vi "Section Page.vi"(8 "error in (no error)":errorcluster, 11 "Node Ptr":T1 format="%.0x") -> (0 "error out":errorcluster)   [LabVIEW 2023, in "J1939 Addon System Explorer.lvlib"]
uses:
  J1939 Addon System Explorer.lvlib
  <vilib>/NI VeriStand/Custom Device API/Custom Device Item Ref.ctl
  Addon Shared/SubVIs/Constants.vi
  <vilib>/NI VeriStand/Custom Device API/Custom Device API.lvlib
  Addon Shared/J1939 Addon Shared.lvlib
panel:
  in  "SHDocVw.IWebBrowser2":refnum<k7>(container)
types:
  T1 = typedef "Custom Device API.lvlib/Custom Device Item Ref.ctl" = u64
  T2 = typedef "Custom Device API.lvlib/Custom Device Item Info.ctl" = cluster{"Name":string, "Is Channel":bool, "GUID":string, "Is Waveform":bool}
  T3 = typedef "Custom Device API.lvlib/Custom Device Commands.ctl" = enum16{"Default", "Item renamed", "Shutdown", "Dynamic button pressed"}
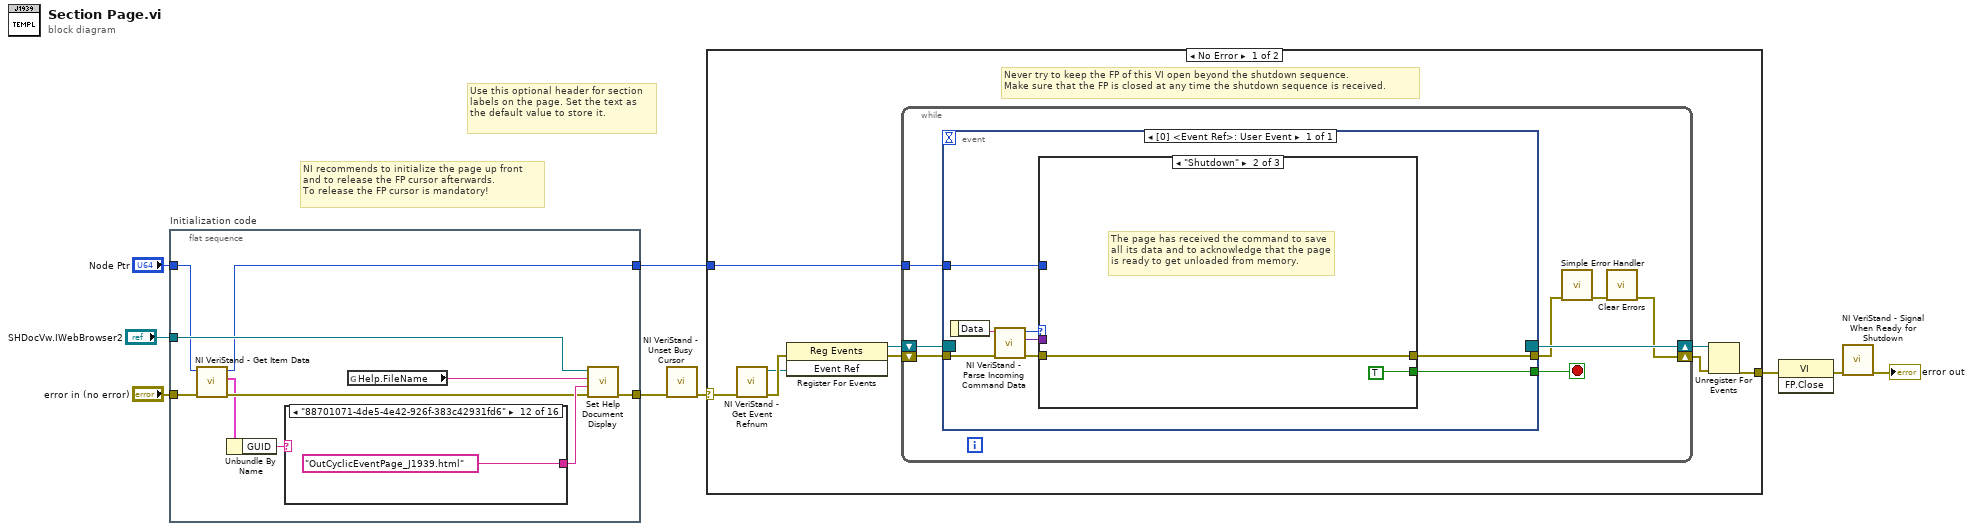
[diagram p0: block diagram]
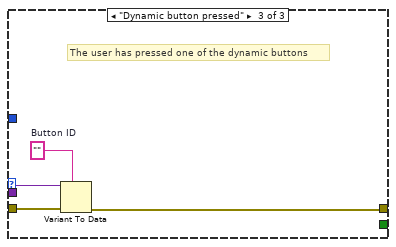
[diagram p3: hidden frame]
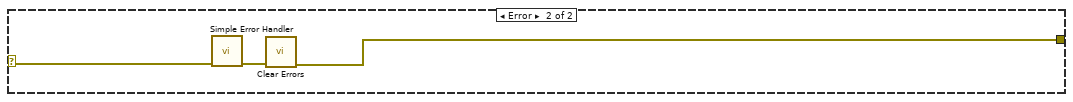
[diagram p4: hidden frame]
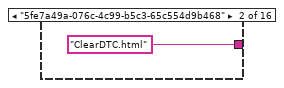
[diagram p6: hidden frame]
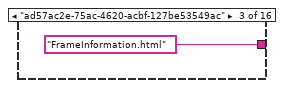
[diagram p7: hidden frame]
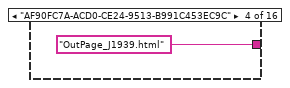
[diagram p8: hidden frame]
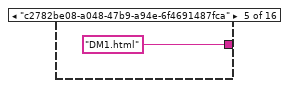
[diagram p9: hidden frame]
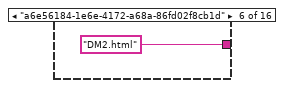
[diagram p10: hidden frame]
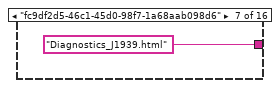
[diagram p11: hidden frame]
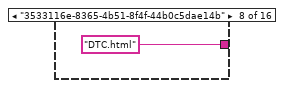
[diagram p12: hidden frame]
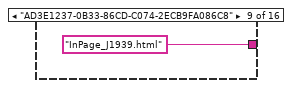
[diagram p13: hidden frame]
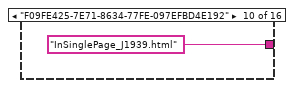
[diagram p14: hidden frame]
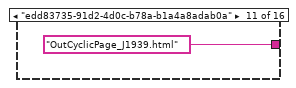
[diagram p15: hidden frame]
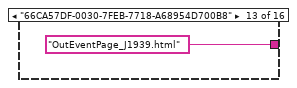
[diagram p16: hidden frame]
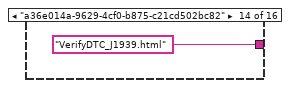
[diagram p17: hidden frame]
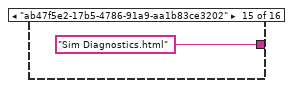
[diagram p18: hidden frame]
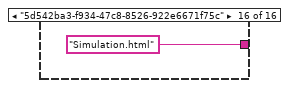
[diagram p19: hidden frame]
diagram:
  # "Use this optional header for section labels on the page. Set the text as the default value to store it."
  # "NI recommends to initialize the page up front\nand to release the FP cursor afterwards.\nTo release the FP cursor is mandatory!"
  n1 = flat-sequence "Initialization code" {
    tunnel: "error in (no error)" -> [w14]
    tunnel: "Node Ptr" -> [w16]
    tunnel: [w18] -> w5
    tunnel: [w15] -> w2
    tunnel: "SHDocVw.IWebBrowser2" -> [w17]
    frame #0 {
      n2 = call <vilib>:"NI VeriStand - Get Item Data.vi"("error in (no error)"=w14, "Item Ref in"=w16) -> ("error out"=w13:errorcluster, "Item Info"=w12:T2, "Item Ref out"=w15:T1)  [unwired: 6 in, 1 out]
      n3 = Unbundle By Name(w12) -> ("GUID"=w11:string)
      n4 = case shown="\"88701071-4de5-4e42-926f-383c42931fd6\"" w11 {
        tunnel: [_ "ClearDTC.html" ("HTML File") "FrameInformation.html" ("HTML File") "OutPage_J1939.html" ("HTML File") "DM1.html" ("HTML File") "DM2.html" ("HTML File") "Diagnostics_J1939.html" ("HTML File") "DTC.html" ("HTML File") "InPage_J1939.html" ("HTML File") "InSinglePage_J1939.html" ("HTML File") "OutCyclicPage_J1939.html" ("HTML File") "OutCyclicEventPage_J1939.html" ("HTML File") "OutEventPage_J1939.html" ("HTML File") "VerifyDTC_J1939.html" ("HTML File") "Sim Diagnostics.html" ("HTML File") "Simulation.html" ("HTML File")] -> w19
        frame Default {
        }
        frame "5fe7a49a-076c-4c99-b5c3-65c554d9b468" {
        }
        frame "ad57ac2e-75ac-4620-acbf-127be53549ac" {
        }
        frame "AF90FC7A-ACD0-CE24-9513-B991C453EC9C" {
        }
        frame "c2782be08-a048-47b9-a94e-6f4691487fca" {
        }
        frame "a6e56184-1e6e-4172-a68a-86fd02f8cb1d" {
        }
        frame "fc9df2d5-46c1-45d0-98f7-1a68aab098d6" {
        }
        frame "3533116e-8365-4b51-8f4f-44b0c5dae14b" {
        }
        frame "AD3E1237-0B33-86CD-C074-2ECB9FA086C8" {
        }
        frame "F09FE425-7E71-8634-77FE-097EFBD4E192" {
        }
        frame "edd83735-91d2-4d0c-b78a-b1a4a8adab0a" {
        }
        frame "88701071-4de5-4e42-926f-383c42931fd6" {
        }
        frame "66CA57DF-0030-7FEB-7718-A68954D700B8" {
        }
        frame "a36e014a-9629-4cf0-b875-c21cd502bc82" {
        }
        frame "ab47f5e2-17b5-4786-91a9-aa1b83ce3202" {
        }
        frame "5d542ba3-f934-47c8-8526-922e6671f75c" {
        }
      }
      n5 = global read "Constants.vi" "Help.FileName"() -> (w10:string)
      n6 = call "Set Help Document Display.vi"("error in (no error)"=w13, "HTML File"=w19, "Main CHM File"=w10, "SHDocVw.IWebBrowser2"=w17) -> ("error out"=w18:errorcluster)  [unwired: 7 in]
    }
  }
  n7 = call <vilib>:"NI VeriStand - Unset Busy Cursor.vi"("error in (no error)"=w5) -> ("error out"=w4:errorcluster)  [unwired: 10 out]
  n8 = case shown="No Error" w4 {
    selector: w4 -> [w35 w69]
    tunnel: [w40 w67] -> w9
    tunnel: w2 -> [w36 _]
    frame No Error {
      # "Never try to keep the FP of this VI open beyond the shutdown sequence.\nMake sure that the FP is closed at any time the shutdown sequence is received."
      n9 = call <vilib>:"NI VeriStand - Get Event Refnum.vi"("error in (no error)"=w35) -> ("error out"=w43:errorcluster, "Event Ref"=w39:refnum<user-event>)  [unwired: 9 out]
      n10 = register-events(error in=w43, w39) -> (reference out=w37:refnum<event-registration>, error out=w38:errorcluster)  [unwired: 1 in]
      n11 = while {
        tunnel: w36 -> [w47]
        shift-right: [w44] -> w41
        shift-left: w38 -> [w50]
        shift-right: [w51] -> w42
        shift-left: w37 -> [w49]
        stop <- w48 stop-if-true
        n12 = event shown="[0] <Event Ref>: User Event" {
          selector: w49 -> [_]
          dyn-events: [_] -> w51
          timeout: _ -> [_]
          tunnel: w50 -> [w59]
          tunnel: [w55] -> w48
          tunnel: [w54] -> w46
          tunnel: w47 -> [w53]
          event User Event {
            n13 = event-data() -> ("Data"=w58:string)  [unwired: 1 out]
            n14 = call <vilib>:"NI VeriStand - Parse Incoming Command Data.vi"("error in (no error)"=w59, "Incoming data"=w58) -> ("error out"=w57:errorcluster, "Outgoing data"=w52:variant, "Action"=w56:T3)  [unwired: 7 out]
            n15 = case shown="\"Shutdown\"" w56 {
              tunnel: w57 -> [w60 w61 w66]
              tunnel: [_ TRUE _] -> w55
              tunnel: [w60 w61 w63] -> w54
              tunnel: w53 -> [_ _ _]
              tunnel: w52 -> [_ _ w65]
              frame "Default", Default {
              }
              frame "Shutdown" {
                # "The page has received the command to save all its data and to acknowledge that the page is ready to get unloaded from memory."
              }
              frame "Dynamic button pressed" {
                w64 = ""  # Button ID
                # "The user has pressed one of the dynamic buttons"
                n16 = Variant To Data(error in=w66, type=w64, Variant=w65) -> (error out=w63:errorcluster)  [unwired: 1 out]
              }
            }
          }
        }
        n17 = call <vilib>:"Simple Error Handler.vi"("error in (no error)"=w46) -> ("error out"=w45:errorcluster)  [unwired: 1 in, 7 out]
        n18 = call <vilib>:"Clear Errors.vi"("error in (no error)"=w45) -> ("error out"=w44:errorcluster)  [unwired: 1 in, 5 out]
      }
      n19 = Unregister For Events(event registration refnum=w42, error in=w41) -> (error out=w40:errorcluster)
    }
    frame Error {
      n20 = call <vilib>:"Simple Error Handler.vi"("error in (no error)"=w69) -> ("error out"=w68:errorcluster)  [unwired: 1 in, 7 out]
      n21 = call <vilib>:"Clear Errors.vi"("error in (no error)"=w68) -> ("error out"=w67:errorcluster)  [unwired: 1 in, 5 out]
    }
  }
  n22 = invoke class="VI" method="FP.Close"(error in=w9) -> (error out=w8:errorcluster)  [unwired: 2 in, 2 out]
  n23 = call <vilib>:"NI VeriStand - Signal When Ready for Shutdown.vi"("error in (no error)"=w8) -> ("error out"=→"error out":errorcluster)  [unwired: 10 out]
